vi "CANOpen_Main_Create xPDO Refs.vi"(8 "error in (no error)":errorcluster, 10 "Nodes":T4[](array[typedef]) {"NMT"."Node init static SDO state" items=["start remote node"=1, "enter pre-operational"=128]; "NMT"."Node run state" items=["start remote node"=1, "stop remote node"=2, "enter pre-operational"=128, "reset node"=129, "reset communication"=130]; "Dynamic SDOs"."Sub-Index (0)" format="%.0x"; "Dynamic SDOs"."Object Index" format="%.0x"; "Dynamic SDOs"."Block Data" format="%.0x"; "RPDOs"."PDO Channel" items=["PDO 1", "PDO 2", "PDO 3", "PDO 4"]; "RPDOs"."Parameters"."Bit Offset" max=8 step=1; "RPDOs"."Parameters"."Byte Offset" max=8 step=1; "TPDOs"."PDO Channel" items=["PDO 1", "PDO 2", "PDO 3", "PDO 4"]; "TPDOs"."Parameters"."Bit Offset" max=8 step=1; "TPDOs"."Parameters"."Byte Offset" max=8 step=1; "SDOs"."Sub-Index (0)" format="%.0x"; "SDOs"."Object Index" format="%.0x"; "SDOs"."Block Data" format="%.0x"}, 11 "interface object":refnum<k20>) -> (0 "error out":errorcluster, 2 "xPDO Refs":T1, 3 "interface object out":refnum<k20>)   [LabVIEW 2021, in "CANOpen Addon Engine.lvlib"]
uses:
  CANOpen Addon Engine.lvlib
  SubVIS/CANOpen_Node Message Settings.ctl
  Shared/CANOpen_PDO Settings.ctl
  Shared/CANOpen_PDO Parameter Settings.ctl
  Shared/CANOpen_PDO Data Type.ctl
  Shared/CANopen Byte Order.ctl
  Shared/CANOpen_SDO Settings.ctl
  SubVIS/CANOpen_NMT Settings.ctl
  Shared/CanOpen_NMT_Config.ctl
  Shared/CanOpen_NMT_Static detect.ctl
  CANOpen_xPDO Refs.ctl
  CanOpen_RPDO Refs.ctl
  CanOpen_TPDO Refs.ctl
  <vilib>/CANopenLib/CANOPEN.llb/CANopen RPDO Create.vi
  <vilib>/CANopenLib/CANOPEN.llb/CANopen TPDO Create.vi
  <resource>/objmgr/CANopenPDO.rc
  Shared/CANOpen Addon Shared.lvlib
panel:
  # "LSB"
  # "MSB"
  # "LSB"
  # "MSB"
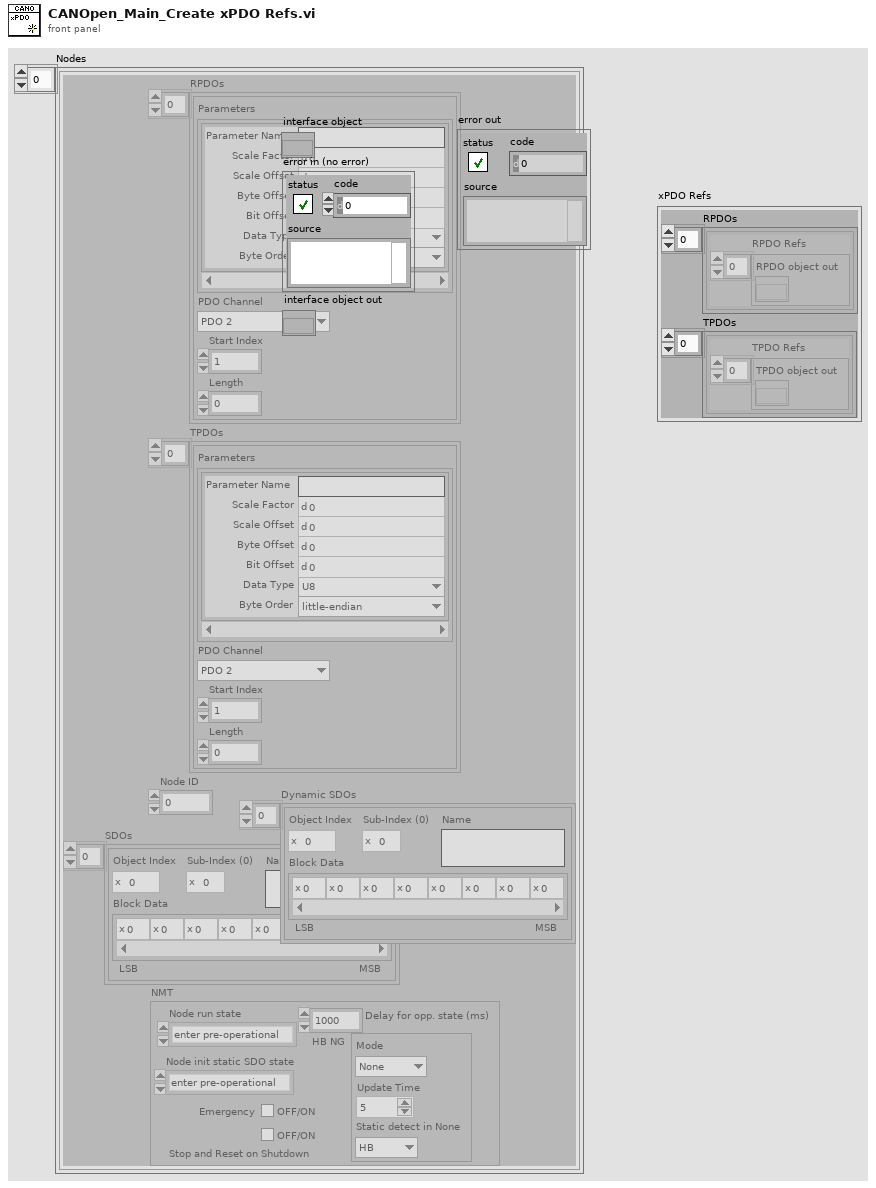
[diagram p1: front panel]
types:
  T1 = typedef "CANOpen Addon Engine.lvlib/CANOpen_xPDO Refs.ctl" = cluster{"RPDOs":T2[], "TPDOs":T3[]}
  T2 = typedef "CANOpen Addon Engine.lvlib/CanOpen_RPDO Refs.ctl" = cluster{"RPDO Refs":refnum<k20>[]}
  T3 = typedef "CANOpen Addon Engine.lvlib/CanOpen_TPDO Refs.ctl" = cluster{"TPDO Refs":refnum<k20>[]}
  T4 = typedef "CANOpen Addon Engine.lvlib/CANOpen_Node Message Settings.ctl" = cluster{"RPDOs":T5[], "TPDOs":T5[], "Node ID":u8, "SDOs":T9[], "Dynamic SDOs":T9[], "NMT":T10}
  T5 = typedef "CANOpen Addon Shared.lvlib/CANOpen_PDO Settings.ctl" = cluster{"Parameters":T6[], "PDO Channel":u8, "Start Index":u32, "Length":u32}
  T6 = typedef "CANOpen Addon Shared.lvlib/CANOpen_PDO Parameter Settings.ctl" = cluster{"Parameter Name":string, "Scale Factor":dbl, "Scale Offset":dbl, "Byte Offset":u8, "Bit Offset":u8, "Data Type":T7, "Byte Order":T8}
  T7 = typedef "CANOpen Addon Shared.lvlib/CANOpen_PDO Data Type.ctl" = enum16{"U8", "U16", "U32", "I8", "I16", "I32", "Single", "Double", "Boolean"}
  T8 = typedef "CANOpen Addon Shared.lvlib/CANopen Byte Order.ctl" = enum16{"big-endian network order", "little-endian"}
  T9 = typedef "CANOpen Addon Shared.lvlib/CANOpen_SDO Settings.ctl" = cluster{"Object Index":u16, "Sub-Index (0)":u8, "Block Data":u8[], "Name":string}
  T10 = typedef "CANOpen Addon Engine.lvlib/CANOpen_NMT Settings.ctl" = cluster{"Node run state":u16, "Emergency":bool, "HB NG":T11, "Delay for opp. state (ms)":dbl, "Node init static SDO state":u16, "Stop and Reset on Shutdown":bool}
  T11 = typedef "CANOpen Addon Shared.lvlib/CanOpen_NMT_Config.ctl" = cluster{"Mode":T12, "Update Time":u16, "Static detect in None":T12}
  T12 = typedef "CANOpen Addon Shared.lvlib/CanOpen_NMT_Static detect.ctl" = enum16{"None", "HB", "NG"}
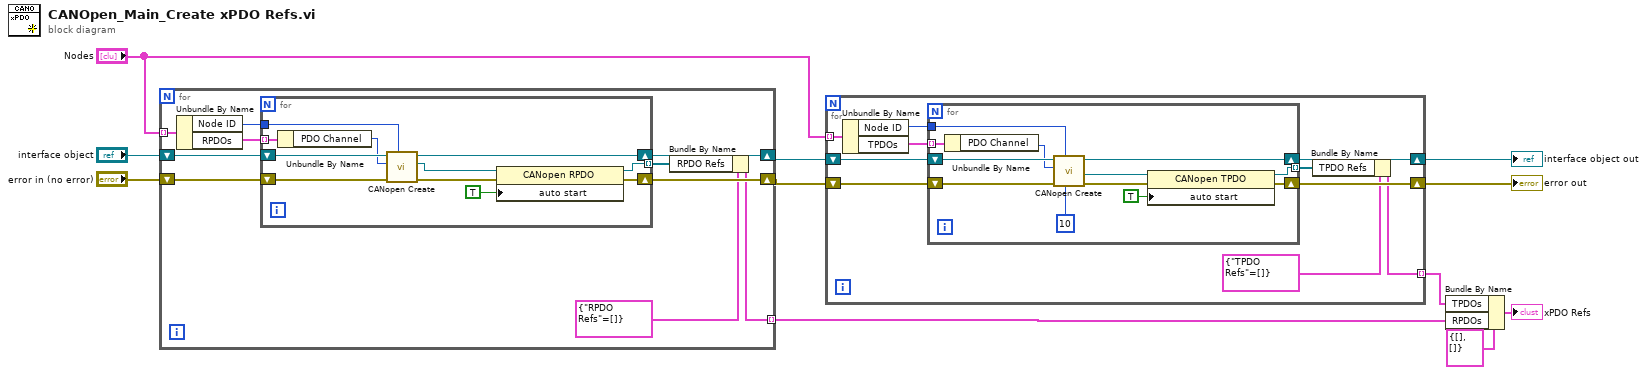
[diagram p0: block diagram]
diagram:
  n1 = for {
    tunnel: [w15] -> w9 mode=indexing
    shift-right: [w20] -> w11
    shift-left: "error in (no error)" -> [w21]
    shift-right: [w12] -> w10
    shift-left: "interface object" -> [w13]
    tunnel: "Nodes" -> [w19] mode=indexing
    n2 = Unbundle By Name(w19) -> ("Node ID"=w18:u8, "RPDOs"=w17:T5[])
    n3 = for {
      tunnel: [w22] -> w16 mode=indexing
      shift-right: [w23] -> w20
      shift-left: w21 -> [w32]
      shift-right: [w27] -> w12
      shift-left: w13 -> [w31]
      tunnel: w18 -> [w30]
      tunnel: w17 -> [w29] mode=indexing
      n4 = Unbundle By Name(w29) -> ("PDO Channel"=w28:u8)
      n5 = call-poly <vilib>:"CANopen Create.vi"("node-ID"=w30, "error in (no error)"=w32, "PDO channel"=w28, "interface object in"=w31) -> ("error out"=w24:errorcluster, "RPDO object out"=w26:refnum<k20>, "interface object out"=w27:refnum<k20>)  [unwired: 5 in]
      n6 = property class="CANopen RPDO"(reference=w26, error in=w24, "auto start"=TRUE) -> (reference out=w22:refnum<k20>, error out=w23:errorcluster)
    }
    n7 = Bundle By Name(cluster=T2 {"RPDO Refs"=[]} ("Node References"), "RPDO Refs"=w16) -> (w15:T2)
  }
  n8 = for {
    tunnel: [w34] -> w7 mode=indexing
    shift-right: [w41] -> w2
    shift-left: w11 -> [w42]
    shift-right: [w40] -> w3
    shift-left: w10 -> [w39]
    tunnel: "Nodes" -> [w38] mode=indexing
    n9 = Unbundle By Name(w38) -> ("Node ID"=w37:u8, "TPDOs"=w36:T5[])
    n10 = for {
      tunnel: [w45] -> w35 mode=indexing
      shift-right: [w49] -> w41
      shift-left: w42 -> [w54]
      shift-right: [w53] -> w40
      shift-left: w39 -> [w52]
      tunnel: w37 -> [w51]
      tunnel: w36 -> [w50] mode=indexing
      n11 = Unbundle By Name(w50) -> ("PDO Channel"=w44:u8)
      n12 = call-poly <vilib>:"CANopen Create.vi"("buffer size (0)"=u16 10, "node-ID"=w51, "error in (no error)"=w54, "PDO channel"=w44, "interface object in"=w52) -> ("error out"=w48:errorcluster, "TPDO object out"=w47:refnum<k20>, "interface object out"=w53:refnum<k20>)  [unwired: 4 in]
      n13 = property class="CANopen TPDO"(reference=w47, error in=w48, "auto start"=TRUE) -> (reference out=w45:refnum<k20>, error out=w49:errorcluster)
    }
    n14 = Bundle By Name(cluster=T3 {"TPDO Refs"=[]} ("Node References"), "TPDO Refs"=w35) -> (w34:T3)
  }
  "error out" <- w2
  "interface object out" <- w3
  n15 = Bundle By Name(cluster=T1 {"RPDOs"=[], "TPDOs"=[]}, "TPDOs"=w7, "RPDOs"=w9) -> (→"xPDO Refs":T1)
